vi "controlGroundAxis.vi"(7 "set":bool, 8 "error in":errorcluster, 9 "groundAxis in":bool, 10 "axis":i32, 11 "connection ID":refnum<k5>) -> (0 "error out":errorcluster, 2 "axis_out":i32, 3 "connection ID":refnum<k5>)   [LabVIEW 2016, in "AMC_VIs.lvlib"]
doc: "Pulls axis piezo drive to GND actively\n only in AMC300\n this is used in MIC-Mode"
uses:
  AMC_VIs.lvlib
panel:
  out "groundAxis out":bool
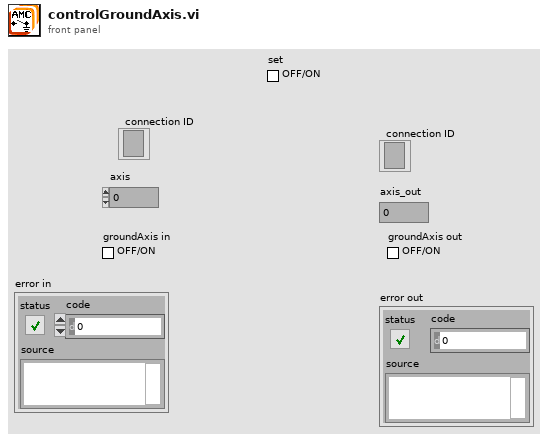
[diagram p1: front panel]
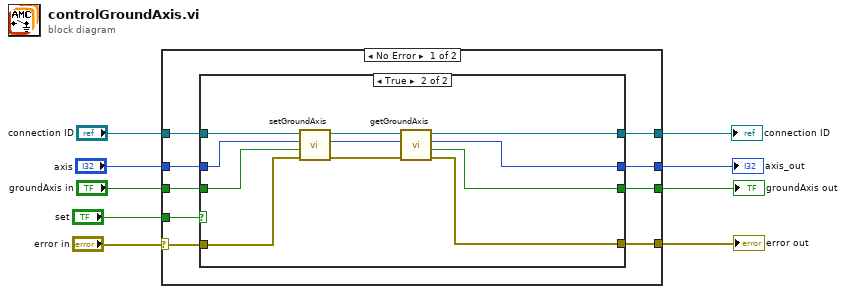
[diagram p0: block diagram]
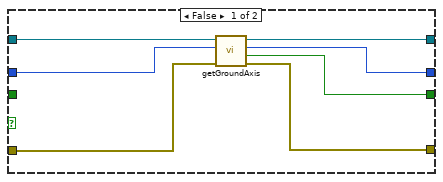
[diagram p2: hidden frame]
diagram:
  n1 = case shown="No Error" "error in" {
    selector: "error in" -> [w15 w40]
    tunnel: [w14 w40] -> w9
    tunnel: [w17 w39] -> w8
    tunnel: "connection ID" -> [w18 w39]
    tunnel: "axis" -> [w13 w37]
    tunnel: "set" -> [w16 _]
    tunnel: "groundAxis in" -> [w12 w38]
    tunnel: [w11 w38] -> w2
    tunnel: [w10 w37] -> w1
    frame No Error {
      n2 = case shown="True" w16 {
        tunnel: w18 -> [w25 w36]
        tunnel: [w24 w26] -> w17
        tunnel: w15 -> [w23 w35]
        tunnel: [w22 w31] -> w14
        tunnel: w13 -> [w20 w34]
        tunnel: w12 -> [_ w33]
        tunnel: [w21 w30] -> w11
        tunnel: [w19 w29] -> w10
        frame False {
          n3 = call "getGroundAxis.vi"("error in"=w23, "axis"=w20, "connection ID"=w25) -> ("error out"=w22:errorcluster, "grounded"=w21:bool, "axis_out"=w19:i32, "connection ID"=w24:refnum<k5>)  [unwired: 5 in]
        }
        frame True {
          n4 = call "setGroundAxis.vi"("error in"=w35, "enabled"=w33, "axis"=w34, "connection ID"=w36) -> ("error out"=w32:errorcluster, "axis_out"=w28:i32, "connection ID"=w27:refnum<k5>)  [unwired: 5 in]
          n5 = call "getGroundAxis.vi"("error in"=w32, "axis"=w28, "connection ID"=w27) -> ("error out"=w31:errorcluster, "grounded"=w30:bool, "axis_out"=w29:i32, "connection ID"=w26:refnum<k5>)  [unwired: 5 in]
        }
      }
    }
    frame Error {
    }
  }
  "error out" <- w9
  "connection ID" <- w8
  "axis_out" <- w1
  "groundAxis out" <- w2
